vi "Sub Create Json File.vi"(8 "error in (no error)":errorcluster, 10 "Json String":string, 11 "Pic Json Generator in":refnum<class "Pic Json Generator.lvclass">) -> (0 "error out":errorcluster, 3 "Pic Json Generator out":refnum<class "Pic Json Generator.lvclass">)   [LabVIEW 2018, in "Pic Json Generator.lvlib" / "Pic Json Generator.lvclass"]
uses:
  Pic Json Generator.lvclass
  Pic Json Generator.lvclass/Pic Json Generator.ctl
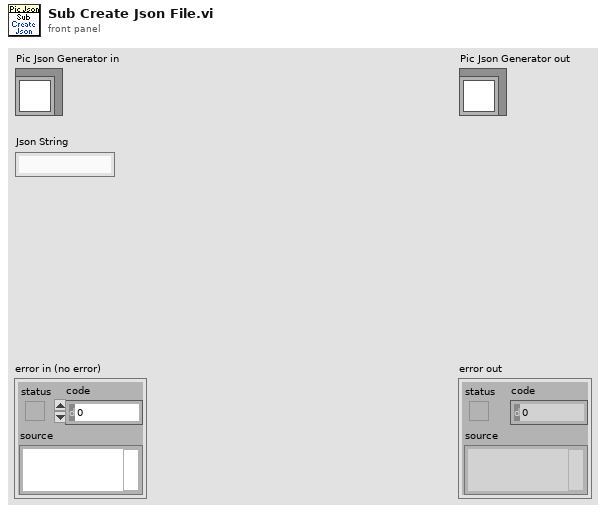
[diagram p1: front panel]
types:
  T1 = enum16{"open", "replace", "create", "open or create", "replace or create", "replace or create with confirmation"}
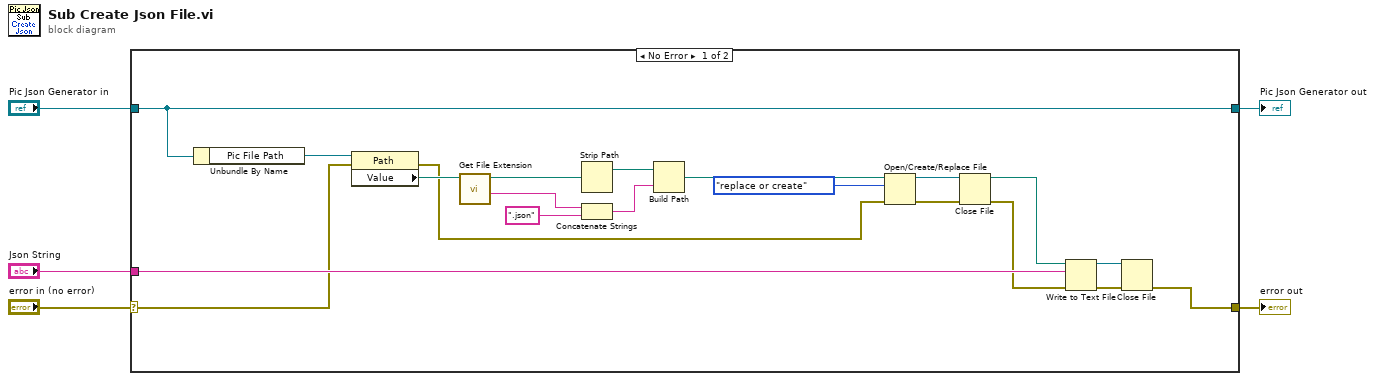
[diagram p0: block diagram]
diagram:
  n1 = case shown="No Error" "error in (no error)" {
    selector: "error in (no error)" -> [w7 w27]
    tunnel: [w6 w27] -> w4
    tunnel: [w25 w26] -> w2
    tunnel: "Pic Json Generator in" -> [w25 w26]
    tunnel: "Json String" -> [w23 _]
    frame No Error {
      n2 = Unbundle By Name(w25) -> ("Pic File Path"=w24:refnum<vi>)
      n3 = property class="Path"(reference=w24, error in=w7) -> (error out=w10:errorcluster, "Value"=w20:path)  [unwired: 1 out]
      n4 = call <vilib>:"Get File Extension.vi"("file"=w20) -> ("filename without extension"=w17:string, "dup file"=w19:path)  [unwired: 6 in, 3 out]
      n5 = Strip Path(path=w19) -> (stripped path=w18:path)  [unwired: 1 out]
      n6 = Concatenate Strings(w17, ".json" ("string")) -> (w15:string)
      n7 = Build Path(base path=w18, name or relative path=w15) -> (appended path=w12:path)
      n8 = Open/Create/Replace File(file path (use dialog)=w12, error in=w10, operation (0:open)=T1."replace or create") -> (refnum out=w14:refnum<file>, error out=w13:errorcluster)  [unwired: 3 in, 1 out]
      n9 = Close File(refnum=w14, error in=w13) -> (path=w8:path, error out=w9:errorcluster)
      n10 = Write to Text File(file (use dialog)=w8, text=w23, error in=w9) -> (refnum out=w22:refnum<file>, error out=w21:errorcluster)  [unwired: 1 in, 1 out]
      n11 = Close File(refnum=w22, error in=w21) -> (error out=w6:errorcluster)  [unwired: 1 out]
    }
    frame Error {
    }
  }
  "error out" <- w4
  "Pic Json Generator out" <- w2
